vi "Convert64BitTo4Channels.vi"(0 "Interleaved Count Array":u64[](array[numeric])) -> (1 "decimated array 0":i16[](array[numeric]), 2 "decimated array 1":i16[](array[numeric]), 3 "decimated array 2":i16[](array[numeric]), 4 "decimated array 3":i16[](array[numeric]))   [LabVIEW 2014]
doc: "Decimates 64 bit count array into 4 count channels."
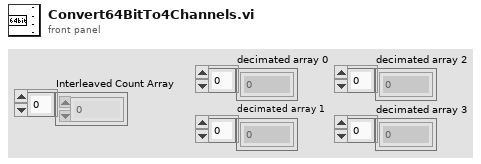
[diagram p1: front panel]
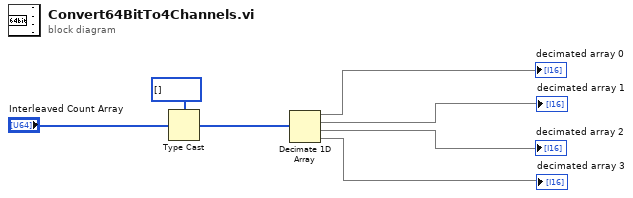
[diagram p0: block diagram]
diagram:
  n1 = Type Cast(type=i16[] [], x="Interleaved Count Array") -> (*(type *) &x=w1:i16[])
  n2 = Decimate 1D Array(w1) -> (→"decimated array 0":i16[], →"decimated array 1":i16[], →"decimated array 2":i16[], →"decimated array 3":i16[])
